vi "MS_test.vi"() -> ()   [LabVIEW 2021]
uses:
  <vilib>/myRIO/Instrument Drivers/Onboard IO/UART/typedef/VISA Configuration.ctl
  <vilib>/Instr/_visa.llb/VISA Configure Serial Port (Instr).vi
  <vilib>/myRIO/Express VI/Onboard IO/UART/UART Express VI.xnode
  <vilib>/myRIO/Instrument Drivers/Onboard IO/UART/UART.lvlib
panel:
  out "Characters Read":string
  in  "stop":bool
  out "number":i32
  out "error out":errorcluster
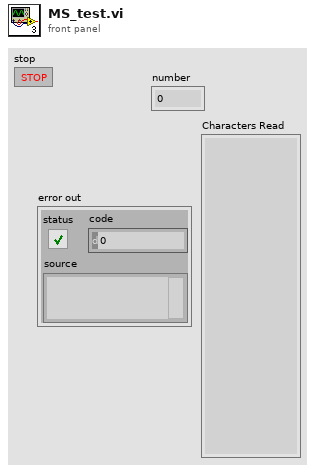
[diagram p1: front panel]
types:
  T1 = typedef "UART.lvlib/VISA Configuration.ctl" = cluster{"baud rate (9600)":u32, "data bits (8)":u16, "parity (0:none)":enum16{"None", "Odd", "Even", "Mark", "Space"}, "stop bits (10: 1 bit)":u16, "flow control (0:none)":u16, "termination char\n(0xA = '\\n' = LF) ":u8, "Enable Termination\nChar (T)":bool, "timeout (10sec)":u32}
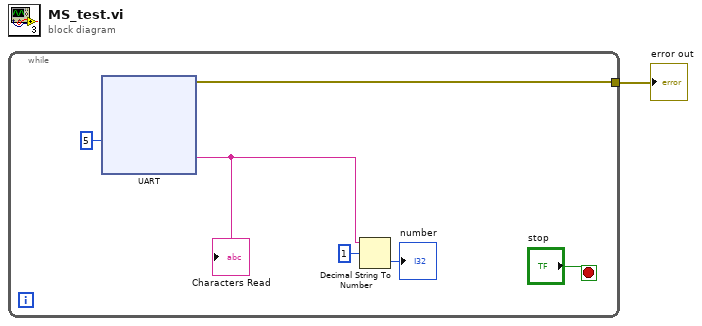
[diagram p0: block diagram]
diagram:
  n1 = while {
    tunnel: [w5] -> w1
    stop <- "stop" stop-if-true
    n2 = xnode "UART"("Character Count"=u32 5) -> ("Characters Read"=w3:string, "error out"=w5:errorcluster)  [unwired: 1 in]
    "Characters Read" <- w3
    n3 = Decimal String To Number(string=w3, offset=1) -> (number=→"number":i32)  [unwired: 1 in, 1 out]
  }
  "error out" <- w1
